vi "Rotate.vi"(8 "Rotation":i32=90, 9 "Direction/Speed":i16=70, 11 "Input":T1) -> (3 "Output":T1)   [LabVIEW 2015]
uses:
  <vilib>/NXT/Subs/LVHSConnector.ctl
  <vilib>/NXT/LegoClasses/BrickReference/BrickReference.lvclass
  <vilib>/NXT/Block Support/NXT_OutputPort.ctl
  <vilib>/NXT/NXTIO Xnodes/NXTIONodeSubVIs/NXTStopMotors.vi
  <vilib>/NXT/Dual Mode Library/Waits/Wait_Num(msec).vi
  <vilib>/NXT/NXTIO Xnodes/NXTIONodeSubVIs/NXTMotorRunDistance.vi
  <vilib>/NXT/NXTIO Xnodes/AddressXNode/NXTIOAddress.xnode
  <vilib>/NXT/NXTIO Xnodes/NXTIOXNode/NXTIO.xnode
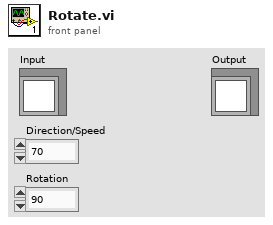
[diagram p1: front panel]
types:
  T1 = typedef "LVHSConnector.ctl" = refnum<class "BrickReference.lvclass">
  T2 = typedef "NXT_OutputPort.ctl" = u8
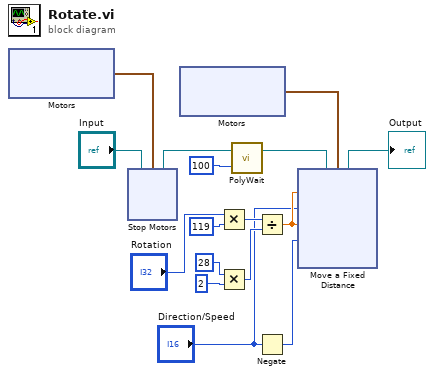
[diagram p0: block diagram]
diagram:
  n1 = xnode "Motors"() -> ("Motor"=w14:cluster{"Port":T2, "Port":T2})
  n2 = xnode "Stop Motors"("Motors"=w14, "NXT/EV3"="Input") -> ("NXT/EV3"=w16:T1)
  n3 = xnode "Motors"() -> ("Motor"=w11:cluster{"Port":T2, "Port":T2})
  n4 = Multiply(x="Rotation", y=119) -> (x*y=w5:i32)
  n5 = Multiply(x=28, y=2) -> (x*y=w6:i32)
  n6 = call-poly <vilib>:"PolyWait.vi"("Time (100 msec)"=u32 100, "NXT/EV3"=w16) -> ("NXT/EV3"=w12:T1)  [unwired: 2 in]
  n7 = Divide(x=w5, y=w6) -> (x/y=w4:dbl)
  n8 = Negate(x="Direction/Speed") -> (-x=w3:i16)
  n9 = xnode "Move a Fixed Distance"("Speed 2"=w3, "Speed 1"="Direction/Speed", "Distance 2"=w4, "Distance 1"=w4, "Motors"=w11, "NXT/EV3"=w12) -> ("NXT/EV3"=→"Output":T1)
